vi "Video File Open.vi"(8 "error in (no error)":errorcluster, 10 "Path":path, 11 "Video File in":refnum<class "Video File.lvclass">) -> (0 "error out":errorcluster, 3 "Video File out":refnum<class "Video File.lvclass">)   [LabVIEW 2018, in "Video File.lvclass"]
uses:
  Video File.lvclass
  <vilib>/vision/Avi.llb/IMAQ AVI2 Codec Path.ctl
  Video File.lvclass/Video File.ctl
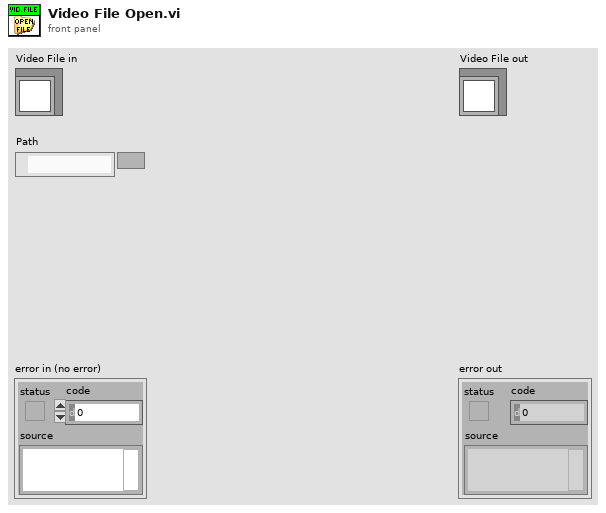
[diagram p1: front panel]
types:
  T1 = typedef "IMAQ AVI2 Codec Path.ctl" = u32
  T2 = typedef "IMAQ AVI2 Refnum.ctl" = refnum<k20>
  T3 = typedef "Image Type" = u32
  T4 = cluster{"Width":u32, "Height":u32, "Frames Per Second":u32, "Codec":string, "Has Data":bool}
  T5 = typedef "IMAQ Image.ctl" = refnum<image>
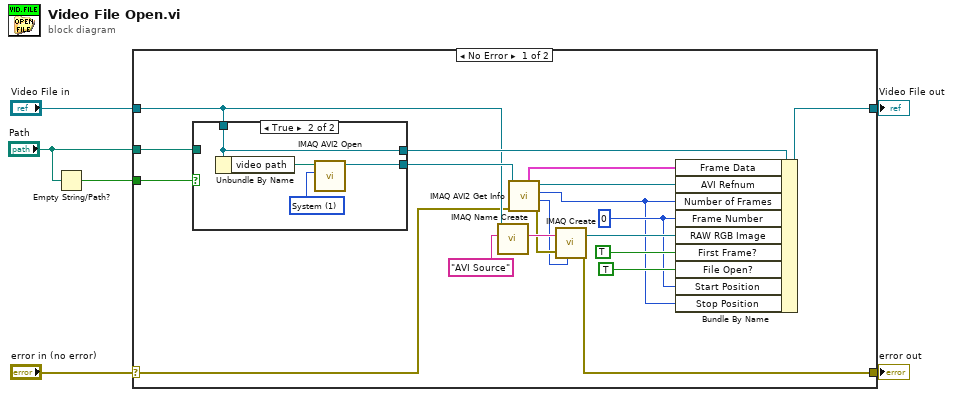
[diagram p0: block diagram]
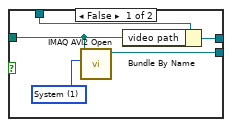
[diagram p2: hidden frame]
diagram:
  n1 = Empty String/Path?(string/path="Path") -> (empty?=w1:bool)
  n2 = case shown="No Error" "error in (no error)" {
    selector: "error in (no error)" -> [w8 w36]
    tunnel: [w13 w36] -> w5
    tunnel: [w12 w35] -> w3
    tunnel: "Video File in" -> [w15 w35]
    tunnel: "Path" -> [w24 _]
    tunnel: w1 -> [w23 _]
    frame No Error {
      w10 = u32 0 ("Frame Number")
      n3 = case shown="True" w23 {
        tunnel: w24 -> [w29 _]
        tunnel: w15 -> [w30 w34]
        tunnel: [w27 w34] -> w22
        tunnel: [w26 w31] -> w21
        frame False {
          w28 = T1 1 items=["Default", "System", "Built in Vision"] ("Codec Source")
          n4 = call "IMAQ AVI2 Open"("Codec Source"=w28, "AVI File Path"=w29) -> ("AVI Refnum"=w26:T2)  [unwired: 1 in, 8 out]
          n5 = Bundle By Name(cluster=w30, "video path"=w29) -> (w27:refnum<class "Video File.lvclass">)
        }
        frame True {
          w33 = T1 1 items=["Default", "System", "Built in Vision"] ("Codec Source")
          n6 = Unbundle By Name(w34) -> ("video path"=w32:path)
          n7 = call "IMAQ AVI2 Open"("Codec Source"=w33, "AVI File Path"=w32) -> ("AVI Refnum"=w31:T2)  [unwired: 1 in, 8 out]
        }
      }
      n8 = call "IMAQ Name Create.vi"("Name (\"\")"="AVI Source" ("Name (\"\")"), "Video File in"=w15) -> ("Name Out"=w16:string)  [unwired: 7 in, 2 out]
      n9 = call "IMAQ AVI2 Get Info"("error in (no error)"=w8, "AVI Refnum"=w21) -> ("error out"=w14:errorcluster, "Image Type"=w7:T3, "Number of Frames"=w9:u32, "AVI Refnum (duplicate)"=w19:T2, "Frame Data"=w20:T4)  [unwired: 5 out]
      n10 = call "IMAQ Create"("Image Name"=w16, "Image Type"=w7, "error in (no error)"=w14) -> ("New Image"=w17:T5, "error out"=w13:errorcluster)  [unwired: 1 in, 1 out]
      n11 = Bundle By Name(cluster=w22, "Frame Data"=w20, "AVI Refnum"=w19, "Number of Frames"=w9, "Frame Number"=w10, "RAW RGB Image"=w17, "First Frame?"=TRUE, "File Open?"=TRUE, "Start Position"=w10, "Stop Position"=w9) -> (w12:refnum<class "Video File.lvclass">)
    }
    frame Error {
    }
  }
  "error out" <- w5
  "Video File out" <- w3
